vi "Simulated Device Page.vi"(8 "error in (no error)":errorcluster, 11 "Node Ptr":T1 format="%.0x") -> (0 "error out":errorcluster)   [LabVIEW 2015, in "J1939 Addon System Explorer.lvlib"]
uses:
  J1939 Addon System Explorer.lvlib
  <vilib>/NI Veristand/Custom Device API/Custom Device Item Ref.ctl
  Shared/Types/Monitor Settings.ctl
  Shared/SubVIs/Constants.vi
  <vilib>/NI Veristand/Custom Device API/Set Item Property (Variant).vi
  <vilib>/NI VeriStand/Custom Device API/Custom Device API.lvlib
  Shared/J1939 Addon Shared.lvlib
panel:
  in  "Settings":cluster{"Section Name":string}={"Section Name"="Address Settings"}
  in  "J1939 Name":u64 format="%.0x"
  in  "J1939 Network Address":u8 format="%.0x"
  in  "Description":string
  in  "Name":string
  in  "SHDocVw.IWebBrowser2":refnum<k7>(container)
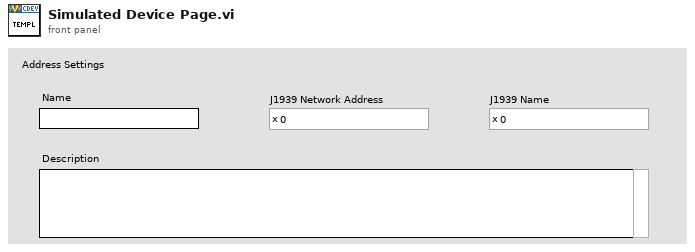
[diagram p1: front panel]
types:
  T1 = typedef "Custom Device API.lvlib/Custom Device Item Ref.ctl" = u64
  T2 = typedef "J1939 Addon Shared.lvlib/Monitor Settings.ctl" = cluster{"Address":u8, "Name":u64}
  T3 = typedef "Custom Device API.lvlib/Custom Device Item Info.ctl" = cluster{"Name":string, "Is Channel":bool, "GUID":string, "Is Waveform":bool}
  T4 = typedef "Custom Device API.lvlib/Custom Device Commands.ctl" = enum16{"Default", "Item renamed", "Shutdown", "Dynamic button pressed"}
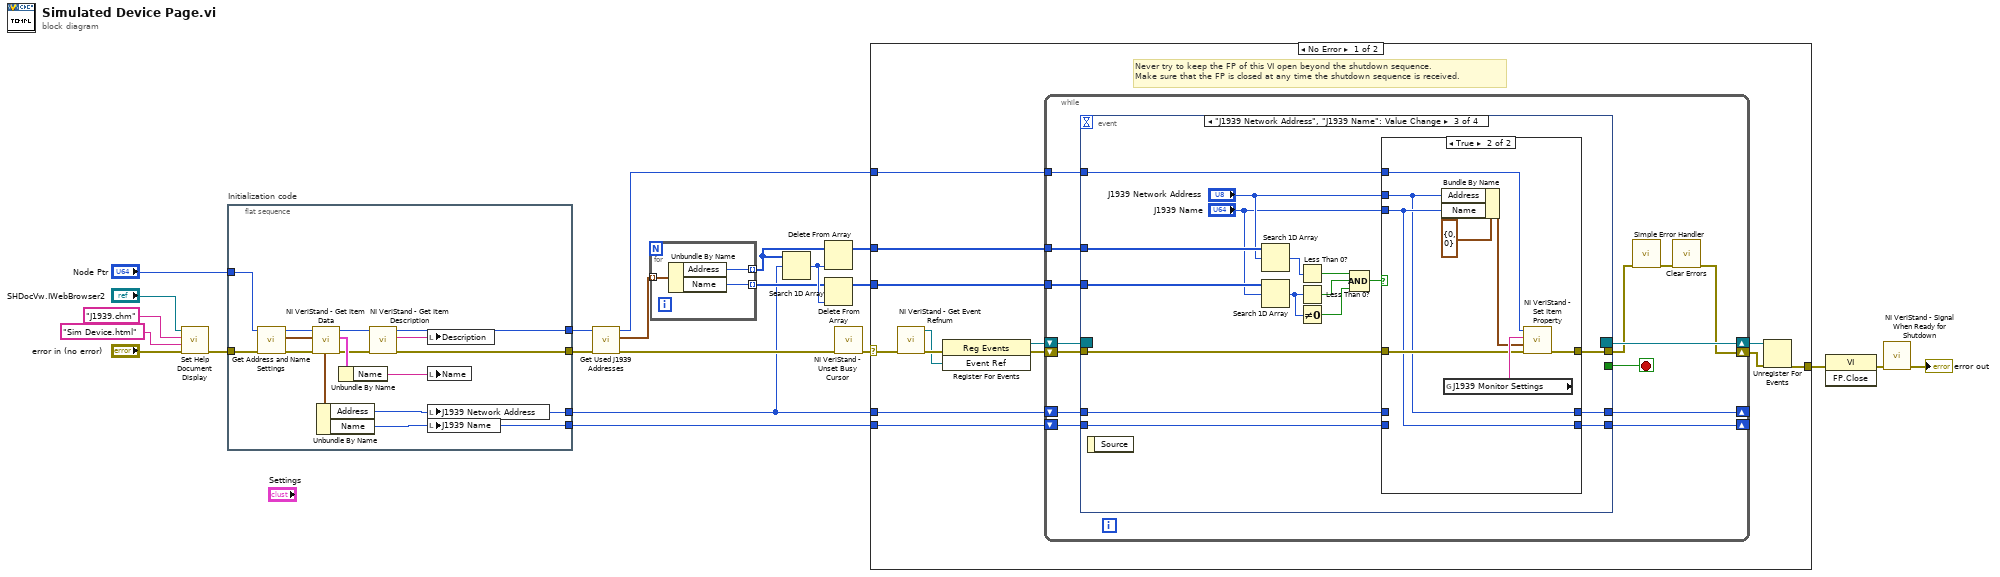
[diagram p0: block diagram]
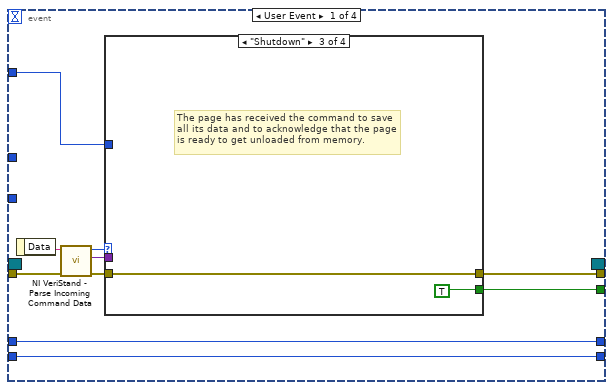
[diagram p2: hidden frame]
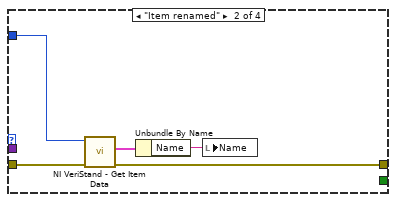
[diagram p4: hidden frame]
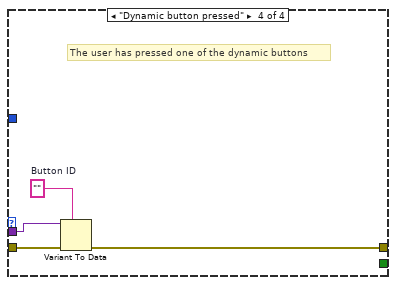
[diagram p5: hidden frame]
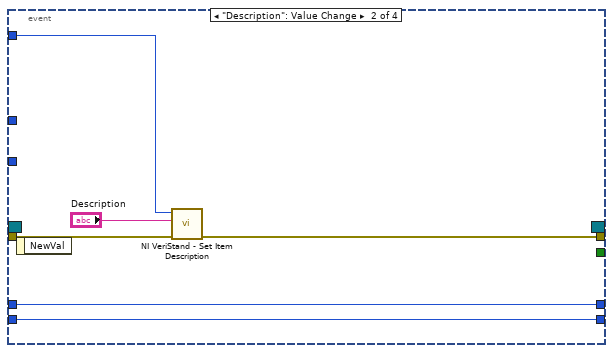
[diagram p6: hidden frame]
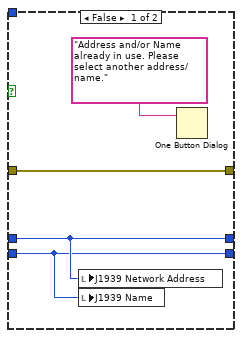
[diagram p7: hidden frame]
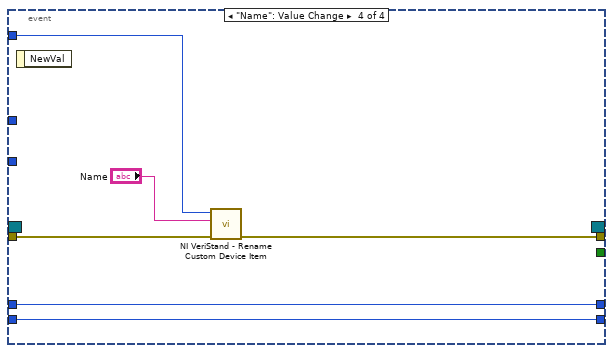
[diagram p8: hidden frame]
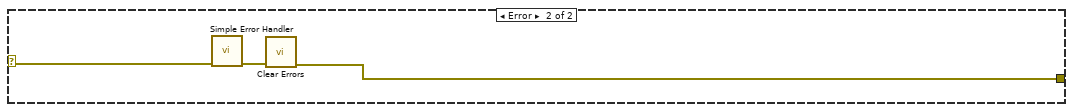
[diagram p9: hidden frame]
diagram:
  n1 = call "Set Help Document Display.vi"("error in (no error)"="error in (no error)", "HTML File"="Sim Device.html", "Main CHM File"="J1939.chm", "SHDocVw.IWebBrowser2"="SHDocVw.IWebBrowser2") -> ("error out"=w13:errorcluster)  [unwired: 7 in]
  n2 = flat-sequence "Initialization code" {
    tunnel: w13 -> [w29]
    tunnel: "Node Ptr" -> [w28]
    tunnel: [w33] -> w11
    tunnel: [w31] -> w9
    tunnel: [w24] -> w3
    tunnel: [w23] -> w8
    frame #0 {
      n3 = call "Get Address and Name Settings.vi"("error in (no error)"=w29, "Node Ref"=w28) -> ("error out"=w26:errorcluster, "J1939 XNET Settings out"=w25:T2, "Node Ref out"=w27:T1)  [unwired: 7 in]
      n4 = call <vilib>:"NI VeriStand - Get Item Data.vi"("error in (no error)"=w26, "Item Ref in"=w27) -> ("error out"=w34:errorcluster, "Item Info"=w36:T3, "Item Ref out"=w32:T1)  [unwired: 7 out]
      n5 = Unbundle By Name(w25) -> ("Address"=w24:u8, "Name"=w23:u64)
      n6 = Unbundle By Name(w36) -> ("Name"=w35:string)
      n7 = call <vilib>:"NI VeriStand - Get Item Description.vi"("error in (no error)"=w34, "Item Ref in"=w32) -> ("error out"=w33:errorcluster, "Description"=w30:string, "Item Ref out"=w31:T1)  [unwired: 6 in, 1 out]
      n8 = local write "Description"(w30) -> ()
      n9 = local write "Name"(w35) -> ()
      n10 = local write "J1939 Network Address"(w24) -> ()
      n11 = local write "J1939 Name"(w23) -> ()
    }
  }
  n12 = call "Get Used J1939 Addresses.vi"("error in (no error)"=w11, "Node Ptr"=w9) -> ("error out"=w12:errorcluster, "Nodes"=w4:T2[], "Item Ref out"=w10:T1)  [unwired: 7 in]
  n13 = for {
    tunnel: w4 -> [w39] mode=indexing
    tunnel: [w38] -> w7 mode=indexing
    tunnel: [w37] -> w5 mode=indexing
    n14 = Unbundle By Name(w39) -> ("Address"=w38:u8, "Name"=w37:u64)
  }
  n15 = Search 1D Array(1D array=w7, element=w3) -> (index of element=w6:i32)  [unwired: 1 in]
  n16 = Delete From Array(array=w7, index=w6) -> (array with subset deleted=w2:u8[])  [unwired: 1 in, 1 out]
  n17 = Delete From Array(array=w5, index=w6) -> (array with subset deleted=w1:u64[])  [unwired: 1 in, 1 out]
  n18 = call <vilib>:"NI VeriStand - Unset Busy Cursor.vi"("error in (no error)"=w12) -> ("error out"=w18:errorcluster)  [unwired: 10 out]
  n19 = case shown="No Error" w18 {
    selector: w18 -> [w44 w132]
    tunnel: [w49 w130] -> w22
    tunnel: w10 -> [w45 _]
    tunnel: w3 -> [w43 _]
    tunnel: w8 -> [w42 _]
    tunnel: w2 -> [w41 _]
    tunnel: w1 -> [w40 _]
    frame No Error {
      # "Never try to keep the FP of this VI open beyond the shutdown sequence.\nMake sure that the FP is closed at any time the shutdown sequence is received."
      n20 = call <vilib>:"NI VeriStand - Get Event Refnum.vi"("error in (no error)"=w44) -> ("error out"=w52:errorcluster, "Event Ref"=w48:refnum<user-event>)  [unwired: 9 out]
      n21 = register-events(error in=w52, w48) -> (reference out=w46:refnum<event-registration>, error out=w47:errorcluster)  [unwired: 1 in]
      n22 = while {
        tunnel: w45 -> [w62]
        shift-right: [w59] -> w50
        shift-left: w47 -> [w65]
        shift-right: [w66] -> w51
        shift-left: w46 -> [w64]
        tunnel: w41 -> [w56]
        tunnel: w40 -> [w55]
        shift-right: [w54] -> _
        shift-left: w43 -> [w58]
        shift-right: [w53] -> _
        shift-left: w42 -> [w57]
        stop <- w63 stop-if-true
        n23 = event shown="[2] \"J1939 Network Address\", \"J1939 Name\": Value Change" {
          selector: w64 -> [_ _ _ _]
          dyn-events: [_ _ _ _] -> w66
          timeout: _ -> [_ _ _ _]
          tunnel: w65 -> [w76 w94 w111 w129]
          tunnel: [w72 _ _ _] -> w63
          tunnel: [w71 w91 w110 w127] -> w61
          tunnel: w62 -> [w70 w92 w109 w128]
          tunnel: w58 -> [w67 w89 w108 w124]
          tunnel: w57 -> [w68 w90 w107 w125]
          tunnel: w56 -> [_ _ w101 _]
          tunnel: w55 -> [_ _ w100 _]
          tunnel: [w67 w89 w96 w124] -> w54
          tunnel: [w68 w90 w95 w125] -> w53
          event User Event {
            n24 = event-data() -> ("Data"=w75:string)  [unwired: 1 out]
            n25 = call <vilib>:"NI VeriStand - Parse Incoming Command Data.vi"("error in (no error)"=w76, "Incoming data"=w75) -> ("error out"=w74:errorcluster, "Outgoing data"=w69:variant, "Action"=w73:T4)  [unwired: 7 out]
            n26 = case shown="\"Shutdown\"" w73 {
              tunnel: w74 -> [w77 w80 w83 w88]
              tunnel: [_ _ TRUE _] -> w72
              tunnel: [w77 w78 w83 w85] -> w71
              tunnel: w70 -> [_ w79 _ _]
              tunnel: w69 -> [_ _ _ w87]
              frame "Default", Default {
              }
              frame "Item renamed" {
                n27 = call <vilib>:"NI VeriStand - Get Item Data.vi"("error in (no error)"=w80, "Item Ref in"=w79) -> ("error out"=w78:errorcluster, "Item Info"=w81:T3)  [unwired: 8 out]
                n28 = Unbundle By Name(w81) -> ("Name"=w82:string)
                n29 = local write "Name"(w82) -> ()
              }
              frame "Shutdown" {
                # "The page has received the command to save all its data and to acknowledge that the page is ready to get unloaded from memory."
              }
              frame "Dynamic button pressed" {
                w86 = ""  # Button ID
                # "The user has pressed one of the dynamic buttons"
                n30 = Variant To Data(error in=w88, type=w86, Variant=w87) -> (error out=w85:errorcluster)  [unwired: 1 out]
              }
            }
          }
          event "Description": Value Change {
            n31 = event-data() -> ()  [unwired: 2 out]
            n32 = call <vilib>:"NI VeriStand - Set Item Description.vi"("error in (no error)"=w94, "Description"="Description", "Item Ref in"=w92) -> ("error out"=w91:errorcluster)  [unwired: 6 in, 2 out]
          }
          event "J1939 Network Address", "J1939 Name": Value Change {
            n33 = event-data() -> ()  [unwired: 2 out]
            n34 = Search 1D Array(1D array=w101, element="J1939 Network Address") -> (index of element=w104:i32)  [unwired: 1 in]
            n35 = Search 1D Array(1D array=w100, element="J1939 Name") -> (index of element=w103:i32)  [unwired: 1 in]
            n36 = Less Than 0?(x=w104) -> (x < 0?=w106:bool)
            n37 = Less Than 0?(x=w103) -> (x < 0?=w105:bool)
            n38 = Not Equal To 0?(x=w103) -> (x != 0?=w102:bool)
            n39 = Compound Arithmetic op=AND(w106, w105, w102) -> (w97:bool)
            n40 = case shown="True" w97 {
              tunnel: "J1939 Name" -> [_ w117]
              tunnel: w111 -> [w115 w121]
              tunnel: [w115 w120] -> w110
              tunnel: w109 -> [_ w119]
              tunnel: "J1939 Network Address" -> [_ w116]
              tunnel: w108 -> [w113 _]
              tunnel: w107 -> [w112 _]
              tunnel: [w113 w116] -> w96
              tunnel: [w112 w117] -> w95
              frame False {
                n41 = local write "J1939 Network Address"(w113) -> ()
                n42 = local write "J1939 Name"(w112) -> ()
                n43 = One Button Dialog(message="Address and/or Name already in use. Please select another address/name.") -> ()  [unwired: 1 in, 1 out]
              }
              frame True {
                n44 = Bundle By Name(cluster=T2 {"Address"=0, "Name"=0} ("J1939 XNET Settings"), "Address"=w116, "Name"=w117) -> (w118:T2)
                n45 = global read "Constants.vi" "J1939 Monitor Settings"() -> (w122:string)
                n46 = call-poly <vilib>:"NI VeriStand - Set Item Property.vi"("error in (no error)"=w121, "Value"=w118, "Property Name"=w122, "Item Ref in"=w119) -> ("error out"=w120:errorcluster)  [unwired: 5 in, 2 out]
              }
            }
          }
          event "Name": Value Change {
            n47 = event-data() -> ()  [unwired: 2 out]
            n48 = call <vilib>:"NI VeriStand - Rename Custom Device Item.vi"("error in (no error)"=w129, "New Name"="Name", "Item Ref in"=w128) -> ("error out"=w127:errorcluster)  [unwired: 1 in, 7 out]
          }
        }
        n49 = call <vilib>:"Simple Error Handler.vi"("error in (no error)"=w61) -> ("error out"=w60:errorcluster)  [unwired: 1 in, 7 out]
        n50 = call <vilib>:"Clear Errors.vi"("error in (no error)"=w60) -> ("error out"=w59:errorcluster)  [unwired: 1 in, 5 out]
      }
      n51 = Unregister For Events(event registration refnum=w51, error in=w50) -> (error out=w49:errorcluster)
    }
    frame Error {
      n52 = call <vilib>:"Simple Error Handler.vi"("error in (no error)"=w132) -> ("error out"=w131:errorcluster)  [unwired: 1 in, 7 out]
      n53 = call <vilib>:"Clear Errors.vi"("error in (no error)"=w131) -> ("error out"=w130:errorcluster)  [unwired: 1 in, 5 out]
    }
  }
  n54 = invoke class="VI" method="FP.Close"(error in=w22) -> (error out=w21:errorcluster)  [unwired: 2 in, 2 out]
  n55 = call <vilib>:"NI VeriStand - Signal When Ready for Shutdown.vi"("error in (no error)"=w21) -> ("error out"=→"error out":errorcluster)  [unwired: 10 out]
